vi "E2_Chicharronera.vi"() -> ()   [LabVIEW 2020]
panel:
  out "x2":cdb
  out "x1":cdb
  in  "c":dbl
  in  "b":dbl
  in  "a":dbl
  out "LED":bool
  out "Nota":string
  out "Resultado":dbl
  in  "Entrada":dbl
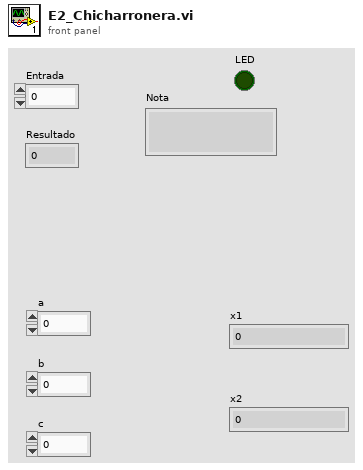
[diagram p1: front panel]
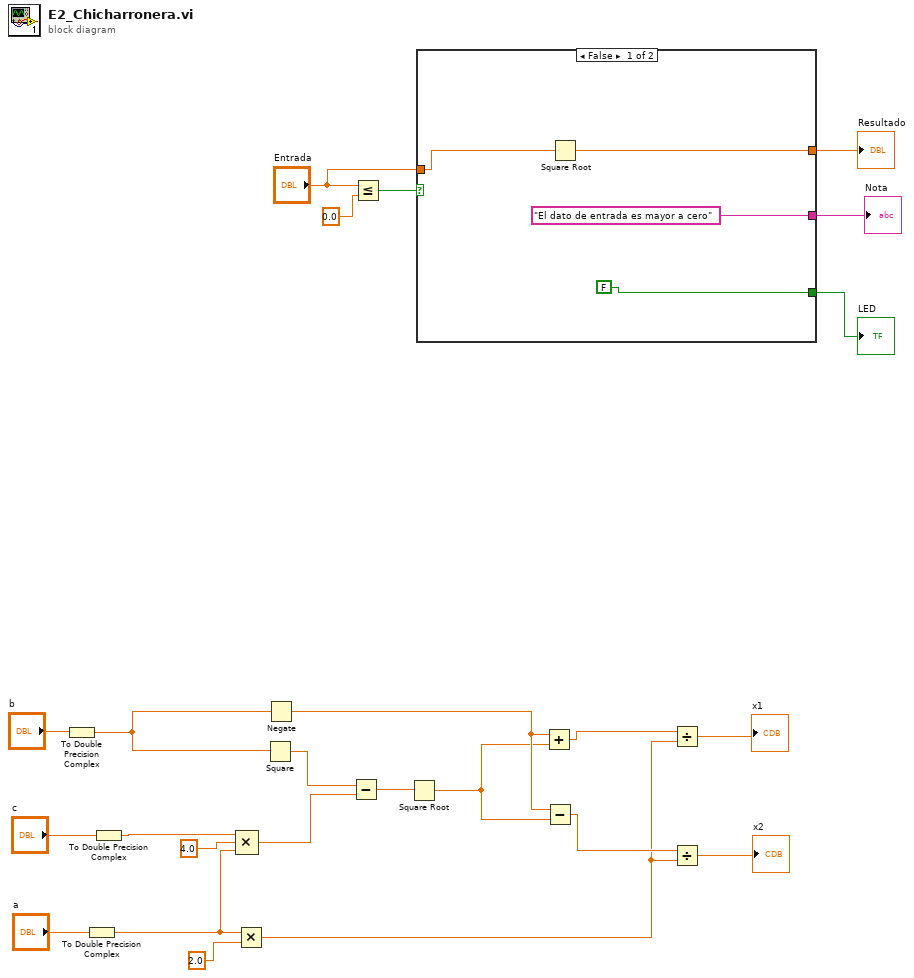
[diagram p0: block diagram]
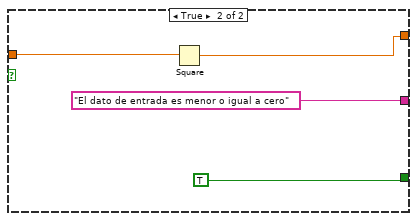
[diagram p2: hidden frame]
diagram:
  n1 = To Double Precision Complex(1:"b") -> (0:w5:cdb)
  n2 = To Double Precision Complex(1:"a") -> (0:w1:cdb)
  n3 = To Double Precision Complex(1:"c") -> (0:w3:cdb)
  n4 = Compound Arithmetic op=MULTIPLY(w3, 4.0 ("value"), w1) -> (w15:cdb)
  n5 = Multiply(x=w1, y=2.0) -> (x*y=w10:cdb)
  n6 = Square(x=w5) -> (x^2=w16:cdb)
  n7 = Negate(x=w5) -> (-x=w13:cdb)
  n8 = Subtract(x=w16, y=w15) -> (x-y=w14:cdb)
  n9 = Less Or Equal?(x="Entrada", y=0.0) -> (x <= y?=w23:bool)
  n10 = Square Root(x=w14) -> (sqrt(x)=w12:cdb)
  n11 = case shown="False" w23 {
    tunnel: "Entrada" -> [w28 w32]
    tunnel: [w27 w31] -> w21
    tunnel: [FALSE TRUE] -> w20
    tunnel: ["El dato de entrada es mayor a cero" "El dato de entrada es menor o igual a cero"] -> w19
    frame False {
      n12 = Square Root(x=w28) -> (sqrt(x)=w27:dbl)
    }
    frame True {
      n13 = Square(x=w32) -> (x^2=w31:dbl)
    }
  }
  "Resultado" <- w21
  "LED" <- w20
  "Nota" <- w19
  n14 = Add(x=w13, y=w12) -> (x+y=w9:cdb)
  n15 = Subtract(x=w13, y=w12) -> (x-y=w11:cdb)
  n16 = Divide(x=w9, y=w10) -> (x/y=→"x1":cdb)
  n17 = Divide(x=w11, y=w10) -> (x/y=→"x2":cdb)
